vi "Drive Turn Left.vi"(7 "Description":string, 8 "Command Info In":T1, 9 "Deadband Value":dbl=0.01, 10 "Right Setpoint":dbl, 11 "Left Setpoint":dbl) -> (0 "Command Info Out":T1)   [LabVIEW 2018]
doc: "This VI notifies the subsystem to the new setpoint."
uses:
  <vilib>/Rock Robotics/WPI/Framework/Command Status Info.ctl
  <vilib>/Rock Robotics/WPI/Framework/Completion Status.ctl
  <vilib>/Rock Robotics/WPI/Framework/Completion Notifier.ctl
  Implementation/Drive Setpoints.ctl
  Implementation/Drive Operations.ctl
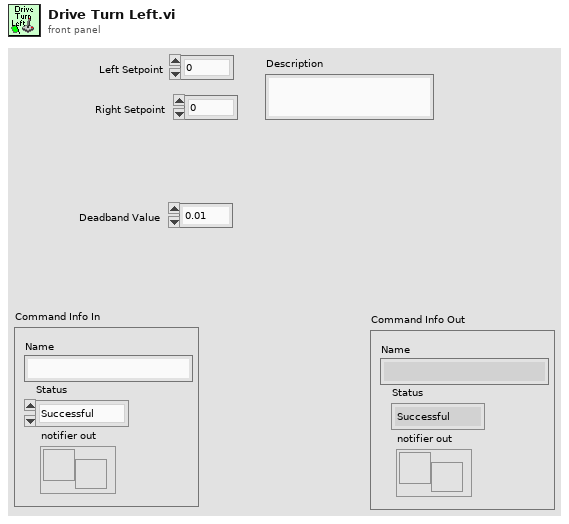
[diagram p1: front panel]
types:
  T1 = typedef "Command Status Info.ctl" = cluster{"Name":string, "Status":T2, "notifier out":T3}
  T2 = typedef "Completion Status.ctl" = enum16{"Successful", "Aborted", "Incomplete"}
  T3 = typedef "Completion Notifier.ctl" = refnum<notifier>
  T4 = typedef "Drive Setpoints.ctl" = cluster{"Operation":T5, "Left Setpoint":dbl, "Right Setpoint":dbl, "Duration":dbl}
  T5 = typedef "Drive Operations.ctl" = enum16{"Reserve", "Read Current", "Immediate", "Drive for Time", "Drive for Distance", "Turn Left", "Turn Right"}
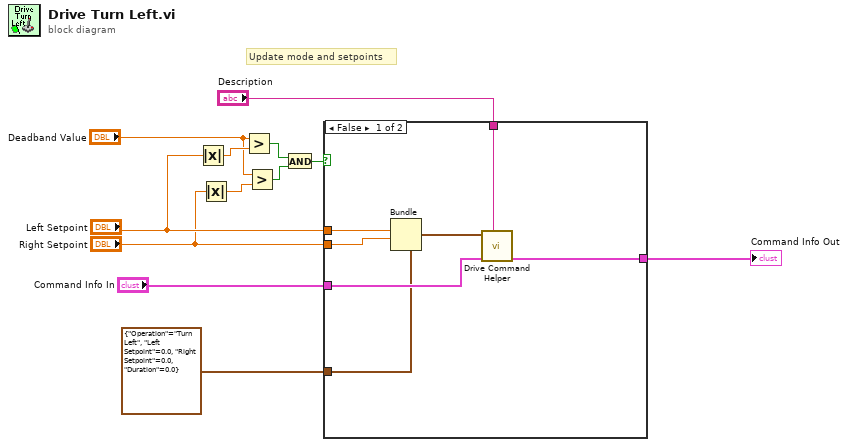
[diagram p0: block diagram]
diagram:
  # "Update mode and setpoints"
  n1 = Absolute Value(x="Left Setpoint") -> (abs(x)=w5:dbl)
  n2 = Absolute Value(x="Right Setpoint") -> (abs(x)=w7:dbl)
  n3 = Greater?(x="Deadband Value", y=w5) -> (0:w6:bool)
  n4 = Greater?(x="Deadband Value", y=w7) -> (0:w8:bool)
  n5 = And(x=w6, y=w8) -> (x .and. y?=w1:bool)
  n6 = case shown="False" w1 {
    tunnel: [w19 w20] -> w12
    tunnel: "Command Info In" -> [w18 w20]
    tunnel: "Description" -> [w17 _]
    tunnel: T4 {"Operation"=enum."Turn Left", "Left Setpoint"=0.0, "Right Setpoint"=0.0, "Duration"=0.0} ("SubSystem Data") -> [w16 _]
    tunnel: "Left Setpoint" -> [w14 _]
    tunnel: "Right Setpoint" -> [w13 _]
    frame False {
      n7 = Bundle(cluster=w16, "Left Setpoint"=w14, "Right Setpoint"=w13) -> (w15:T4)  [unwired: 2 in]
      n8 = call "Drive Command Helper.vi"("Description"=w17, "Command Info In"=w18, "SubSystem Data"=w15) -> ("Command Info Out"=w19:T1)  [unwired: 6 in, 2 out]
    }
    frame True {
    }
  }
  "Command Info Out" <- w12
